vi "Register Message.vi"(8 "error in (no error)":errorcluster, 10 "TestManagerMsg":refnum<class "TestManagerMsg.lvclass">, 11 "Basic Test Manager in":refnum<class "Basic Test Manager.lvclass">) -> (0 "error out":errorcluster, 3 "Basic Test Manager out":refnum<class "Basic Test Manager.lvclass">)   [LabVIEW 2013, in "Caraya.lvlib" / "Basic Test Manager.lvclass"]
uses:
  Basic Test Manager.lvclass
  Test Manager Message/TestManagerMsg.lvclass
  Basic Test Manager.lvclass/Basic Test Manager.ctl
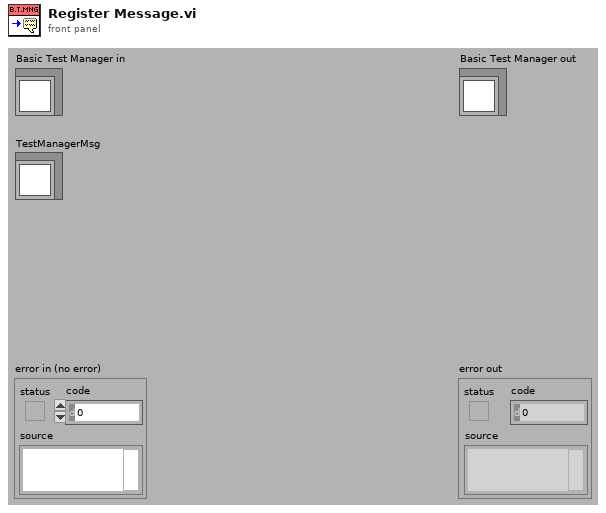
[diagram p1: front panel]
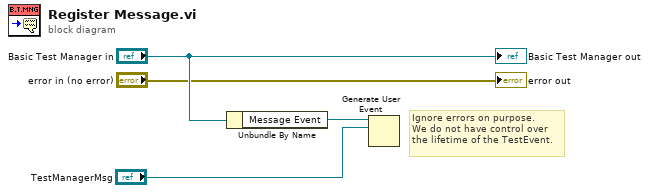
[diagram p0: block diagram]
diagram:
  # "Ignore errors on purpose.\nWe do not have control over\nthe lifetime of the TestEvent."
  n1 = Unbundle By Name("Basic Test Manager in") -> ("Message Event"=w2:refnum<user-event>)
  n2 = Generate User Event(user event=w2, event data cluster="TestManagerMsg") -> ()  [unwired: 2 in, 2 out]
  "error out" <- "error in (no error)"
  "Basic Test Manager out" <- "Basic Test Manager in"
